vi "Pusher_Client_Utility_StopFG.vi"(7 "Command":enum16{"Write", "Read", "Reset"}(ring)=enum."Read", 8 "error in (no error)":errorcluster, 10 "Stop on Error?":bool, 11 "Stop?":bool) -> (0 "error out":errorcluster, 2 "Latched Stop":bool, 5 "OnError?":bool)   [LabVIEW 2009, in "Client.lvclass"]
uses:
  Client.lvclass
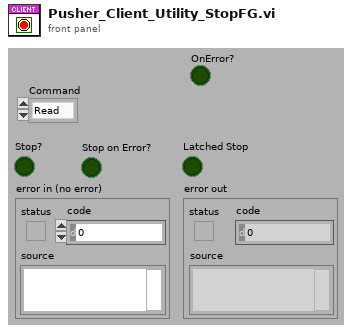
[diagram p1: front panel]
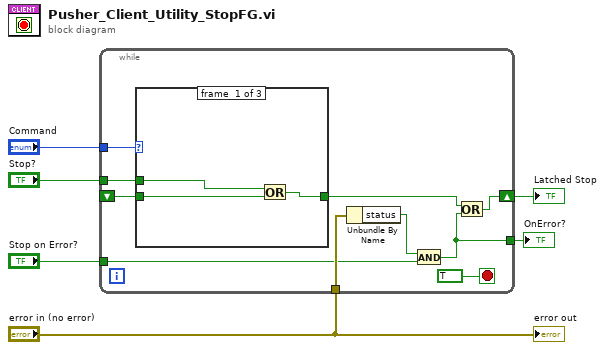
[diagram p0: block diagram]
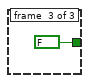
[diagram p3: hidden frame]
diagram:
  n1 = while {
    shift-right: [w12] -> w3
    shift-left: _ -> [w15]
    tunnel: "Stop?" -> [w14]
    tunnel: "Command" -> [w13]
    tunnel: "error in (no error)" -> [w10]
    tunnel: "Stop on Error?" -> [w8]
    tunnel: [w7] -> w1
    stop <- TRUE stop-if-true
    n2 = case shown="\"Reset\"" w13 {
      tunnel: w15 -> [w19 w20 _]
      tunnel: [w17 w20 FALSE ("Stop?")] -> w11
      tunnel: w14 -> [w18 _ _]
      frame #0 {
        n3 = Or(x=w18, y=w19) -> (x .or. y?=w17:bool)
      }
      frame #1 {
      }
      frame #2 {
      }
    }
    n4 = Unbundle By Name(w10) -> ("status"=w9:bool)
    n5 = And(x=w9, y=w8) -> (x .and. y?=w7:bool)
    n6 = Or(x=w11, y=w7) -> (x .or. y?=w12:bool)
  }
  "Latched Stop" <- w3
  "OnError?" <- w1
  "error out" <- "error in (no error)"
